vi "Start 1Hz livestream video from CamServer (TCP CLIENT).vi"(4 "Quality":i32=750 min=0 max=1000, 6 "Resolution":T1 items=["Low", "Med.", "High", "Max."], 7 "Camera":T3="Travcam", 8 "Video name":string, 9 "Video directory path":path, 10 "Write video":bool, 11 "TCP/IP port":u16=80) -> (0 "Error out":errorcluster)   [LabVIEW 2015]
doc: "Starts a video livestream from the camera server. The stream can also be saved to a local directory."
uses:
  Camera enum/Camera enum.ctl
  Camera enum/Camera resolution.ctl
  <vilib>/vision/Avi.llb/IMAQ AVI2 Refnum.ctl
  Globals/CamServer global.vi
panel:
  in  "Stop":bool
  out "Video":T2(plugin-control)
  # "PN 01/09/15"
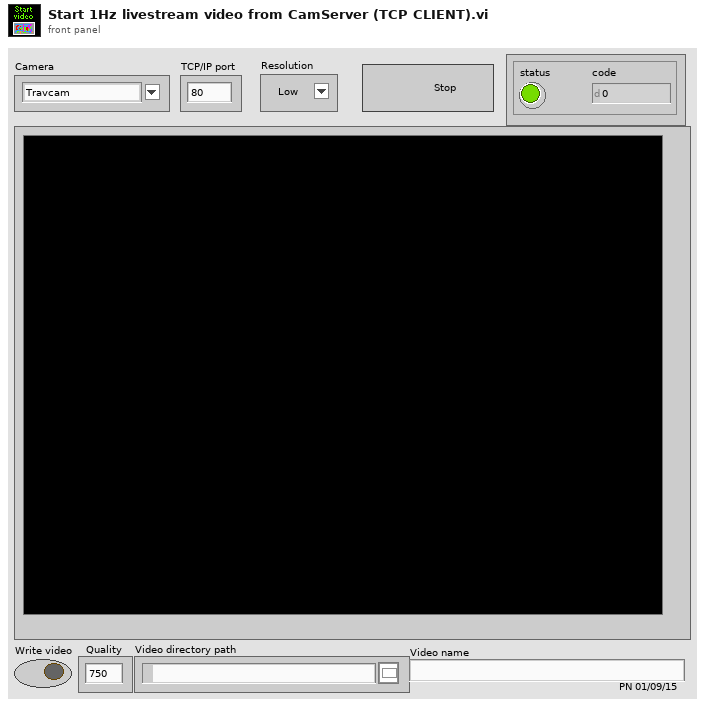
[diagram p1: front panel]
types:
  T1 = typedef "Camera resolution.ctl" = u8
  T2 = typedef "IMAQ Image.ctl" = refnum<image>
  T3 = typedef "Camera enum.ctl" = string
  T4 = typedef "IMAQ AVI2 Refnum.ctl" = refnum<k20>
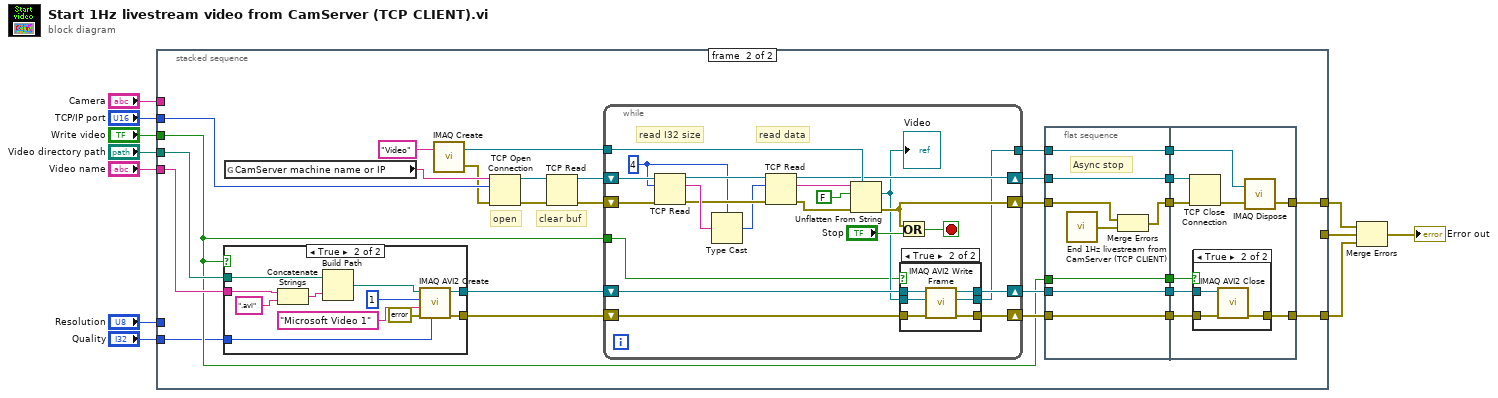
[diagram p0: block diagram]
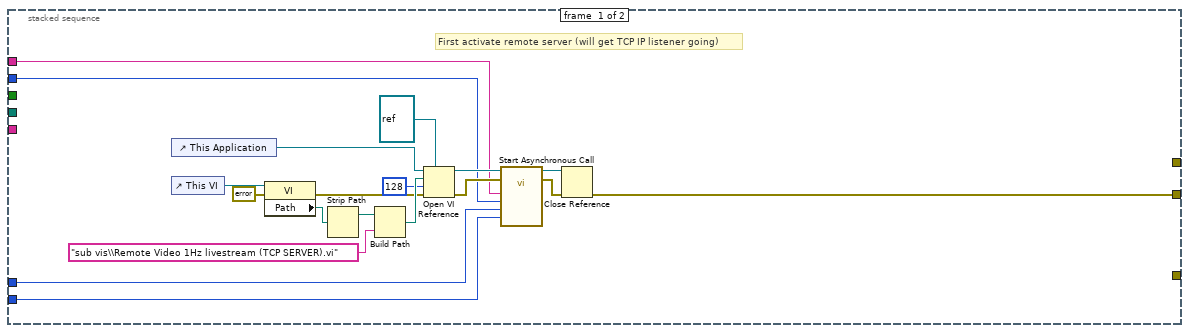
[diagram p2: hidden frame]
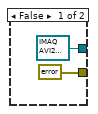
[diagram p3: hidden frame]
diagram:
  n1 = stacked-sequence {
    tunnel: "Camera" -> [w16 _]
    tunnel: "TCP/IP port" -> [w15 w58]
    tunnel: "Write video" -> [_ w33]
    tunnel: [w14 _] -> w8
    tunnel: [_ w43] -> w7
    tunnel: [_ w36] -> w5
    tunnel: "Video name" -> [_ w35]
    tunnel: "Video directory path" -> [_ w34]
    tunnel: "Quality" -> [w13 w31]
    tunnel: "Resolution" -> [w12 _]
    frame #0 {
      # "First activate remote server (will get TCP IP listener going)"
      n2 = control-ref of="This Application"() -> (w25:refnum<vi>)
      n3 = control-ref of="This VI"() -> (w30:refnum<vi>)
      n4 = property class="VI"(reference=w30, error in=errorcluster {"status"=FALSE, "code"=0, "source"=""} ("error in (no error)")) -> (error out=w27:errorcluster, "Path"=w23:path)  [unwired: 1 out]
      n5 = Strip Path(path=w23) -> (stripped path=w22:path)  [unwired: 1 out]
      n6 = Build Path(base path=w22, name or relative path="sub vis\\Remote Video 1Hz livestream (TCP SERVER).vi") -> (appended path=w28:path)
      n7 = Open VI Reference(type specifier VI Refnum (for type only)=refnum<vi> refnum, application reference (local)=w25, vi path=w28, options=128, error in (no error)=w27) -> (vi reference=w21:refnum<vi>, error out=w20:errorcluster)  [unwired: 1 in]
      n8 = call-by-ref "Start Asynchronous Call"(reference=w21, error in=w20, "Quality"=w13, "Resolution"=w12, "TCP/IP port"=w15, "Camera"=w16) -> (reference out=w18:refnum<vi>, error out=w17:errorcluster)  [unwired: 1 out]
      n9 = Close Reference(reference=w18, error in (no error)=w17) -> (error out=w14:errorcluster)
    }
    frame #1 {
      # "open"
      # "clear buf"
      n10 = case shown="True" w33 {
        tunnel: [T4 refnum ("AVI Refnum") w71] -> w42
        tunnel: [errorcluster {"status"=FALSE, "code"=0, "source"=""} ("error out") w70] -> w41
        tunnel: w35 -> [_ w63]
        tunnel: w34 -> [_ w62]
        tunnel: w31 -> [_ w61]
        frame False {
        }
        frame True {
          n11 = Concatenate Strings(w63, ".avi" ("name or relative path")) -> (w65:string)
          n12 = Build Path(base path=w62, name or relative path=w65) -> (appended path=w64:path)
          n13 = call "IMAQ AVI2 Create"("Quality"=w61, "error in (no error)"=errorcluster {"status"=FALSE, "code"=0, "source"=""} ("error in"), "Codec"="Microsoft Video 1", "Frames Per Second"=u32 1, "AVI Path"=w64) -> ("error out"=w70:errorcluster, "AVI Refnum"=w71:T4)  [unwired: 5 in]
        }
      }
      n14 = global read "CamServer global.vi" "CamServer machine name or IP"() -> (w57:string)
      n15 = call "IMAQ Create"("Image Name"="Video") -> ("New Image"=w51:T2, "error out"=w50:errorcluster)  [unwired: 4 in]
      n16 = TCP Open Connection(address=w57, remote port or service name=w58, error in (no error)=w50) -> (connection ID=w55:refnum<k5>, error out=w56:errorcluster)  [unwired: 2 in]
      n17 = TCP Read(connection ID=w55, error in (no error)=w56) -> (connection ID out=w53:refnum<k5>, error out=w54:errorcluster)  [unwired: 3 in, 1 out]
      n18 = while {
        shift-right: [w103] -> w49
        shift-left: w53 -> [w114]
        shift-right: [w102] -> w48
        shift-left: w54 -> [w112]
        tunnel: w51 -> [w105]
        tunnel: [w93] -> w47
        shift-right: [w97] -> w37
        shift-left: w41 -> [w96]
        shift-right: [w98] -> w40
        shift-left: w42 -> [w99]
        tunnel: w33 -> [w94]
        stop <- w100 stop-if-true
        w104 = 4
        # "read data"
        # "read I32 size"
        n19 = TCP Read(connection ID=w114, bytes to read=w104, error in (no error)=w112) -> (connection ID out=w111:refnum<k5>, data out=w113:string, error out=w110:errorcluster)  [unwired: 2 in]
        n20 = Type Cast(type=w104, x=w113) -> (*(type *) &x=w109:i32)
        n21 = TCP Read(connection ID=w111, bytes to read=w109, error in (no error)=w110) -> (connection ID out=w103:refnum<k5>, data out=w108:string, error out=w106:errorcluster)  [unwired: 2 in]
        n22 = Unflatten From String(type=w105, binary string=w108, data includes array or string size? (T)=FALSE, error in (no error)=w106) -> (value=w95:T2, error out=w102:errorcluster)  [unwired: 1 in, 1 out]
        "Video" <- w95
        n23 = Or(x=w102, y="Stop") -> (x .or. y?=w100:bool)
        n24 = case shown="True" w94 {
          tunnel: w99 -> [w117 w123]
          tunnel: w95 -> [w115 w122]
          tunnel: [w117 w121] -> w98
          tunnel: [w116 w120] -> w97
          tunnel: w96 -> [w116 w119]
          tunnel: [w115 w118] -> w93
          frame False {
          }
          frame True {
            n25 = call "IMAQ AVI2 Write Frame"("error in (no error)"=w119, "Image"=w122, "AVI Refnum"=w123) -> ("error out"=w120:errorcluster, "Image Out (duplicate)"=w118:T2, "AVI Refnum (duplicate)"=w121:T4)  [unwired: 6 in]
          }
        }
      }
      n26 = flat-sequence {
        tunnel: w47 -> [w78]
        tunnel: w48 -> [w76]
        tunnel: w49 -> [w79]
        tunnel: [w79] -> w46
        tunnel: [w75] -> w45
        tunnel: [w78] -> w44
        tunnel: w40 -> [w74]
        tunnel: [w74] -> w39
        tunnel: w37 -> [w73]
        tunnel: [w73] -> w38
        tunnel: w33 -> [w72]
        tunnel: [w72] -> w32
        tunnel: w46 -> [w88]
        tunnel: w45 -> [w87]
        tunnel: w44 -> [w85]
        tunnel: [w84] -> w43
        tunnel: w39 -> [w83]
        tunnel: w38 -> [w82]
        tunnel: [w81] -> w36
        tunnel: w32 -> [w80]
        frame #0 {
          # "Async stop"
          n27 = call "End 1Hz livestream from CamServer (TCP CLIENT).vi"() -> ("Error out"=w77:errorcluster)  [unwired: 1 in]
          n28 = Merge Errors(w76, w77) -> (w75:errorcluster)
        }
        frame #1 {
          n29 = TCP Close Connection(connection ID=w88, error in (no error)=w87) -> (error out=w86:errorcluster)  [unwired: 1 in, 1 out]
          n30 = case shown="True" w80 {
            tunnel: w82 -> [w89 w92]
            tunnel: [w89 w91] -> w81
            tunnel: w83 -> [_ w90]
            frame False {
            }
            frame True {
              n31 = call "IMAQ AVI2 Close"("error in (no error)"=w92, "AVI Refnum"=w90) -> ("error out"=w91:errorcluster)  [unwired: 9 in]
            }
          }
          n32 = call "IMAQ Dispose"("Image"=w85, "error in (no error)"=w86) -> ("error out"=w84:errorcluster)  [unwired: 4 in]
        }
      }
    }
  }
  n33 = Merge Errors(w7, w8, w5) -> (→"Error out":errorcluster)
